vi "get_selected_ROI.vi"(8 "error in (no error)":errorcluster, 11 "RoiCollection in":refnum<class "RoiCollection.lvclass">) -> (0 "error out":errorcluster, 1 "ID of currently selected ROI":string, 2 "RoiGeneric.lvclass":refnum<class "RoiGeneric.lvclass">, 3 "RoiCollection out":refnum<class "RoiCollection.lvclass">, 4 "any ROI selected?":bool)   [LabVIEW 2010, in "RoiCollection.lvclass"]
uses:
  RoiCollection.lvclass
  RoiGeneric/RoiGeneric.lvclass
  RoiCollection.lvclass/RoiCollection.ctl
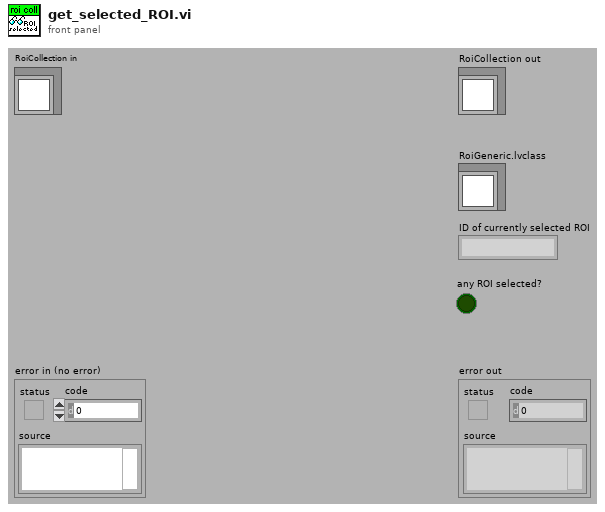
[diagram p1: front panel]
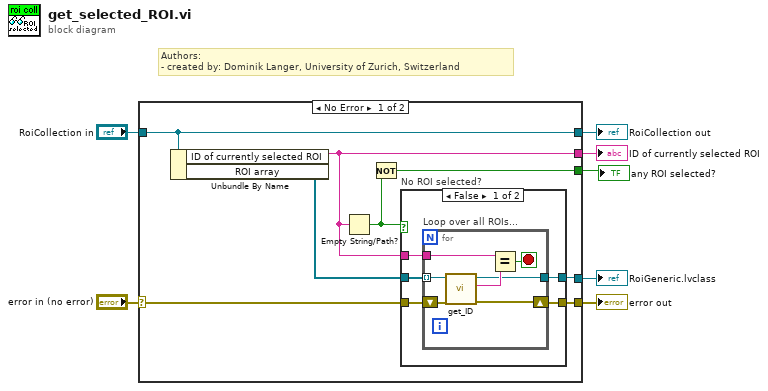
[diagram p0: block diagram]
diagram:
  # "Authors: \n- created by: Dominik Langer, University of Zurich, Switzerland"
  n1 = case shown="No Error" "error in (no error)" {
    selector: "error in (no error)" -> [w13 w30]
    tunnel: [w12 w30] -> w6
    tunnel: [w15 w29] -> w4
    tunnel: "RoiCollection in" -> [w15 w29]
    tunnel: [w10 _] -> w3
    tunnel: [w11 _] -> w2
    tunnel: [w8 _] -> w1
    frame No Error {
      n2 = Unbundle By Name(w15) -> ("ID of currently selected ROI"=w10:string, "ROI array"=w14:refnum<class "RoiGeneric.lvclass">[])
      n3 = Empty String/Path?(string/path=w10) -> (empty?=w9:bool)
      n4 = Not(x=w9) -> (.not. x?=w8:bool)
      n5 = case "No ROI selected?" shown="False" w9 {
        tunnel: w14 -> [w20 _]
        tunnel: w13 -> [w19 w28]
        tunnel: [w18 w28] -> w12
        tunnel: [w17 _] -> w11
        tunnel: w10 -> [w16 _]
        frame False {
          n6 = for "Loop over all ROIs..." {
            tunnel: w20 -> [w27] mode=indexing
            shift-right: [w25] -> w18
            shift-left: w19 -> [w26]
            tunnel: w16 -> [w23]
            tunnel: [w21] -> w17
            stop <- w22 stop-if-true
            n7 = call-dynamic "get_ID.vi"("error in (no error)"=w26, "RoiGeneric in"=w27) -> ("error out"=w25:errorcluster, "ID"=w24:string, "RoiGeneric out"=w21:refnum<class "RoiGeneric.lvclass">)  [unwired: 7 in]
            n8 = Equal?(x=w23, y=w24) -> (x = y?=w22:bool)
          }
        }
        frame True {
        }
      }
    }
    frame Error {
    }
  }
  "error out" <- w6
  "RoiCollection out" <- w4
  "RoiGeneric.lvclass" <- w2
  "ID of currently selected ROI" <- w3
  "any ROI selected?" <- w1
